vi "Measurement Logic.vi"(8 "error in":errorcluster, 9 "measurement configuration":T2={"Automation Test"=FALSE, "Power sequencing file path"="", "SMU name"="", "SMU channel"="0", "RFSG name"="5842_0", "RFSG port"="", "RFSG attenuation mode"=enum."Constant Attenuation", "RFSG external attenuation (dB)"=2.0, "RFSG s-parameters orientation"=enum."Port2 Towards DUT", "RFSG s2p file path"="", "RFmx name"="5842_0", "RFmx port"="", "RFmx attenuation mode"=enum."Constant Attenuation", "RFmx external attenuation (dB)"=1.2, "RFmx attenuation path name"="", "RFmx s-parameters orientation"=enum."Port2 Towards DUT", "RFmx attenuation s2p path name"="", "RFmx s2p file path"="", "Compression_Expected DUT Gain (dB)"=17.5, "Compression_Max Linear Range (dBm)"=-10.0, "Compression_Compression Point (dB)"=1.0, "Compression_Target Pin (dBm)"=1.0, "Compression_RFSG Frequency Start (Hz)"=10000000000.0, "Compression_RFSG Frequency Stop (Hz)"=18000000000.0, "Compression_RFSG Number of Frequency Step"=10, "Compression_RFSG Power Start (dBm)"=-20.0, "Compression_RFSG Power Stop(dBm)"=1.0, "Compression_RFSG Power Step Size (dB)"=4.0, "Compression_RBW (Hz)"=0.0, "Compression_RF Measurement Interval (s)"=0.0, "Compression_DC Measurement Interval (s)"=0.001, "Compression_Stimulus Mode"=enum."Constant Power and RF", "CP_CW_DC Source Delay (s)"=0.0, "CP_PRF_DC Source Delay (s)"=0.0, "CP_PRF_RFmx Trigger Delay (s)"=0.0, "CP_PRF_RF Pulse Width (s)"=0.0001, "CP_PRF_PRI (s)"=0.001, "PP_PRF_DC Source Delay (s)"=0.0, "PP_PRF_RFmx Trigger Delay (s)"=0.0, "PP_PRF_RF Pulse Width (s)"=0.0001, "PP_PRF_PRI (s)"=0.001, "PP_PRF_DC Pulse Width (s)"=0.0008, "PP_PRF_ON Current Limit (A)"=2.0, "PP_PRF_Bias Voltage Level (V)"=0.0, "PP_PRF_Bias Current Limit (A)"=0.2} {"Compression_Target Pin (dBm)" format="%#pdBm"; "PP_PRF_Bias Current Limit (A)" format="%#pA"; "PP_PRF_Bias Voltage Level (V)" format="%#pV"; "PP_PRF_ON Current Limit (A)" format="%#pA"; "PP_PRF_DC Pulse Width (s)" format="%#ps"; "PP_PRF_PRI (s)" format="%#ps"; "PP_PRF_RF Pulse Width (s)" format="%#ps"; "PP_PRF_RFmx Trigger Delay (s)" format="%#ps"; "PP_PRF_DC Source Delay (s)" format="%#ps"; "CP_PRF_PRI (s)" format="%#ps"; "CP_PRF_RF Pulse Width (s)" format="%#ps"; "CP_PRF_RFmx Trigger Delay (s)" format="%#ps"; "CP_PRF_DC Source Delay (s)" format="%#ps"; "CP_CW_DC Source Delay (s)" format="%#ps"; "Compression_DC Measurement Interval (s)" format="%#ps"; "Compression_RF Measurement Interval (s)" format="%#ps"; "RFmx external attenuation (dB)" format="%.2f"; "RFSG external attenuation (dB)" format="%.2f"}, 10 "measure call context in":refnum<class "Measure Call Context.lvclass">) -> (0 "error out":errorcluster, 1 "measurement results":T1, 2 "measure call context out":refnum<class "Measure Call Context.lvclass">)   [LabVIEW 2023, in "FPT_Compression.lvclass"]
doc: "Contains the core logic for executing the measurement."
uses:
  FPT_Compression.lvclass
  <vilib>/Plug-In SDKs/Measurements/Measure Call Context/Measure Call Context.lvclass
  Measurement Configuration.ctl
  Measurement Results.ctl
  <vilib>/Analysis/baseanly.llb/Mean (DBL).vi
  <extravilib>/ChannelInstances/Event Messenger-bool/Instantiate.vi
  <vilib>/Analysis/NI_AALBase.lvlib
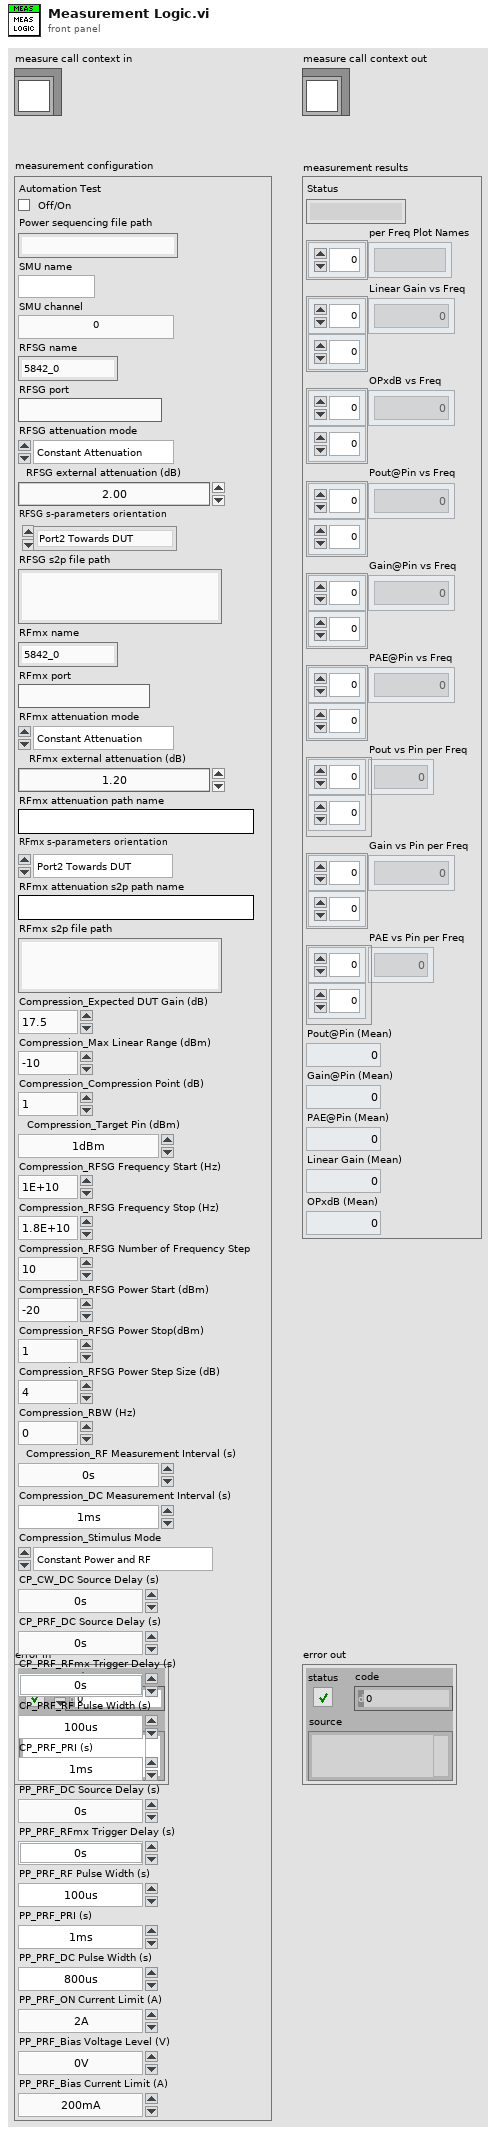
[diagram p1: front panel]
types:
  T1 = typedef "FPT_Compression.lvclass/Measurement Results.ctl" = cluster{"Status":string, "per Freq Plot Names":string[], "Linear Gain vs Freq":dbl[][], "OPxdB vs Freq":dbl[][], "Pout@Pin vs Freq":dbl[][], "Gain@Pin vs Freq":dbl[][], "PAE@Pin vs Freq":dbl[][], "Pout vs Pin per Freq":dbl[][], "Gain vs Pin per Freq":dbl[][], "PAE vs Pin per Freq":dbl[][], "Pout@Pin (Mean)":dbl, "Gain@Pin (Mean)":dbl, "PAE@Pin (Mean)":dbl, "Linear Gain (Mean)":dbl, "OPxdB (Mean)":dbl}
  T2 = typedef "FPT_Compression.lvclass/Measurement Configuration.ctl" = cluster{"Automation Test":bool, "Power sequencing file path":string, "SMU name":string, "SMU channel":string, "RFSG name":string, "RFSG port":string, "RFSG attenuation mode":enum32{"<None>", "Constant Attenuation", "s2p File"}, "RFSG external attenuation (dB)":dbl, "RFSG s-parameters orientation":enum32{"Port1 Towards DUT", "Port2 Towards DUT"}, "RFSG s2p file path":string, "RFmx name":string, "RFmx port":string, "RFmx attenuation mode":enum32{"<None>", "Constant Attenuation", "s2p File"}, "RFmx external attenuation (dB)":dbl, "RFmx attenuation path name":string, "RFmx s-parameters orientation":enum32{"Port1 Towards DUT", "Port2 Towards DUT"}, "RFmx attenuation s2p path name":string, "RFmx s2p file path":string, "Compression_Expected DUT Gain (dB)":dbl, "Compression_Max Linear Range (dBm)":dbl, "Compression_Compression Point (dB)":dbl, "Compression_Target Pin (dBm)":dbl, "Compression_RFSG Frequency Start (Hz)":dbl, "Compression_RFSG Frequency Stop (Hz)":dbl, "Compression_RFSG Number of Frequency Step":i32, "Compression_RFSG Power Start (dBm)":dbl, "Compression_RFSG Power Stop(dBm)":dbl, "Compression_RFSG Power Step Size (dB)":dbl, "Compression_RBW (Hz)":dbl, "Compression_RF Measurement Interval (s)":dbl, "Compression_DC Measurement Interval (s)":dbl, "Compression_Stimulus Mode":enum32{"Constant Power and RF", "Constant Power and Pulsed RF", "Pulsed Power and RF"}, "CP_CW_DC Source Delay (s)":dbl, "CP_PRF_DC Source Delay (s)":dbl, "CP_PRF_RFmx Trigger Delay (s)":dbl, "CP_PRF_RF Pulse Width (s)":dbl, "CP_PRF_PRI (s)":dbl, "PP_PRF_DC Source Delay (s)":dbl, "PP_PRF_RFmx Trigger Delay (s)":dbl, "PP_PRF_RF Pulse Width (s)":dbl, "PP_PRF_PRI (s)":dbl, "PP_PRF_DC Pulse Width (s)":dbl, "PP_PRF_ON Current Limit (A)":dbl, "PP_PRF_Bias Voltage Level (V)":dbl, "PP_PRF_Bias Current Limit (A)":dbl}
  T3 = enum32{"Power On Dut", "De-embedding + Measurement", "Power Off Dut"}[]
  T4 = cluster{"measurement configuration":T2, "measurement results":T1}
  T5 = typedef "RFmx Config - Compression.ctl" = cluster{"RFmx Name":refnum<k15>, "RFmx Port":string, "Attenuation":cluster{"Mode":enum32{"<None>", "Constant Attenuation", "s2p File"}, "Constant Attenuation":cluster{"RFmx External Attenuation (dB)":dbl}, "s2p File":cluster{"RFmx S-Parameters Orientation":i32, "RFmx Attenuation s2p File":path}}}
  T6 = typedef "RFSG Config - Compression.ctl" = cluster{"RFSG Name":refnum<k15>, "RFSG Port":string, "Attenuation":cluster{"Mode":enum32{"<None>", "Constant Attenuation", "s2p File"}, "Contant Attenuation":cluster{"RFSG External Attenuation (dB)":dbl}, "s2p File":cluster{"RFSG S-parameters Orientation":i32, "RFSG s2p File Path":path}}}
  T7 = typedef "Test Config - Compression.ctl" = cluster{"Expected DUT Gain (dB)":dbl, "Max Linear Range (dBm)":dbl, "Compression Point (dB)":dbl, "Pout at Pin (dBm)":dbl, "RFSG Frequency Start (Hz)":dbl, "RFSG Frequency Stop (Hz)":dbl, "RFSG Number of Frequency Step":i32, "Power Start (dBm)":dbl, "Power Stop(dBm)":dbl, "Power Step Size (dB)":dbl, "RBW (Hz)":dbl, "Modes":cluster{"RF Measurement Interval (s)":dbl, "DC Measurement Interval (s)":dbl, "Power Stimulus Mode":enum16{"Constant Power and RF", "Constant Power and Pulsed RF", "Pulsed Power and RF"}, "CP_CW_DC Source Delay (s)":dbl, "CP_PRF_RF Pulse Width (s)":dbl, "CP_PRF_PRI (s)":dbl, "CP_PRF_DC Source Delay (s)":dbl, "CP_PRF_RFmx Trigger Delay (s)":dbl, "PP_PRF_RF Pulse Width (s)":dbl, "PP_PRF_PRI (s)":dbl, "PP_PRF_DC Pulse Width (s)":dbl, "PP_PRF_Bias Voltage Level (V)":dbl, "PP_PRF_Bias Current Limit (A)":dbl, "PP_PRF_DC Source Delay (s)":dbl, "PP_PRF_RFmx Trigger Delay (s)":dbl}}
  T8 = typedef "SMU Config - Compression.ctl" = cluster{"SMU Name":refnum<k15>, "SMU Channel":string, "IDD Current Limit (A)":dbl}
  T9 = typedef "Results - Compression.ctl" = cluster{"Linear Gain vs Freq":dbl[][], "OPxdb vs Freq":dbl[][], "Pout@Pin vs Freq":dbl[][], "Gain@Pin vs Freq":dbl[][], "PAE@Pin vs Freq":dbl[][], "Pout vs Pin per Freq":dbl[][], "Gain vs Pin per Freq":dbl[][], "PAE vs Pin per Freq":dbl[][]}
  T10 = typedef "Event Messenger-bool.lvlib/))Channel.ctl" = refnum<queue>
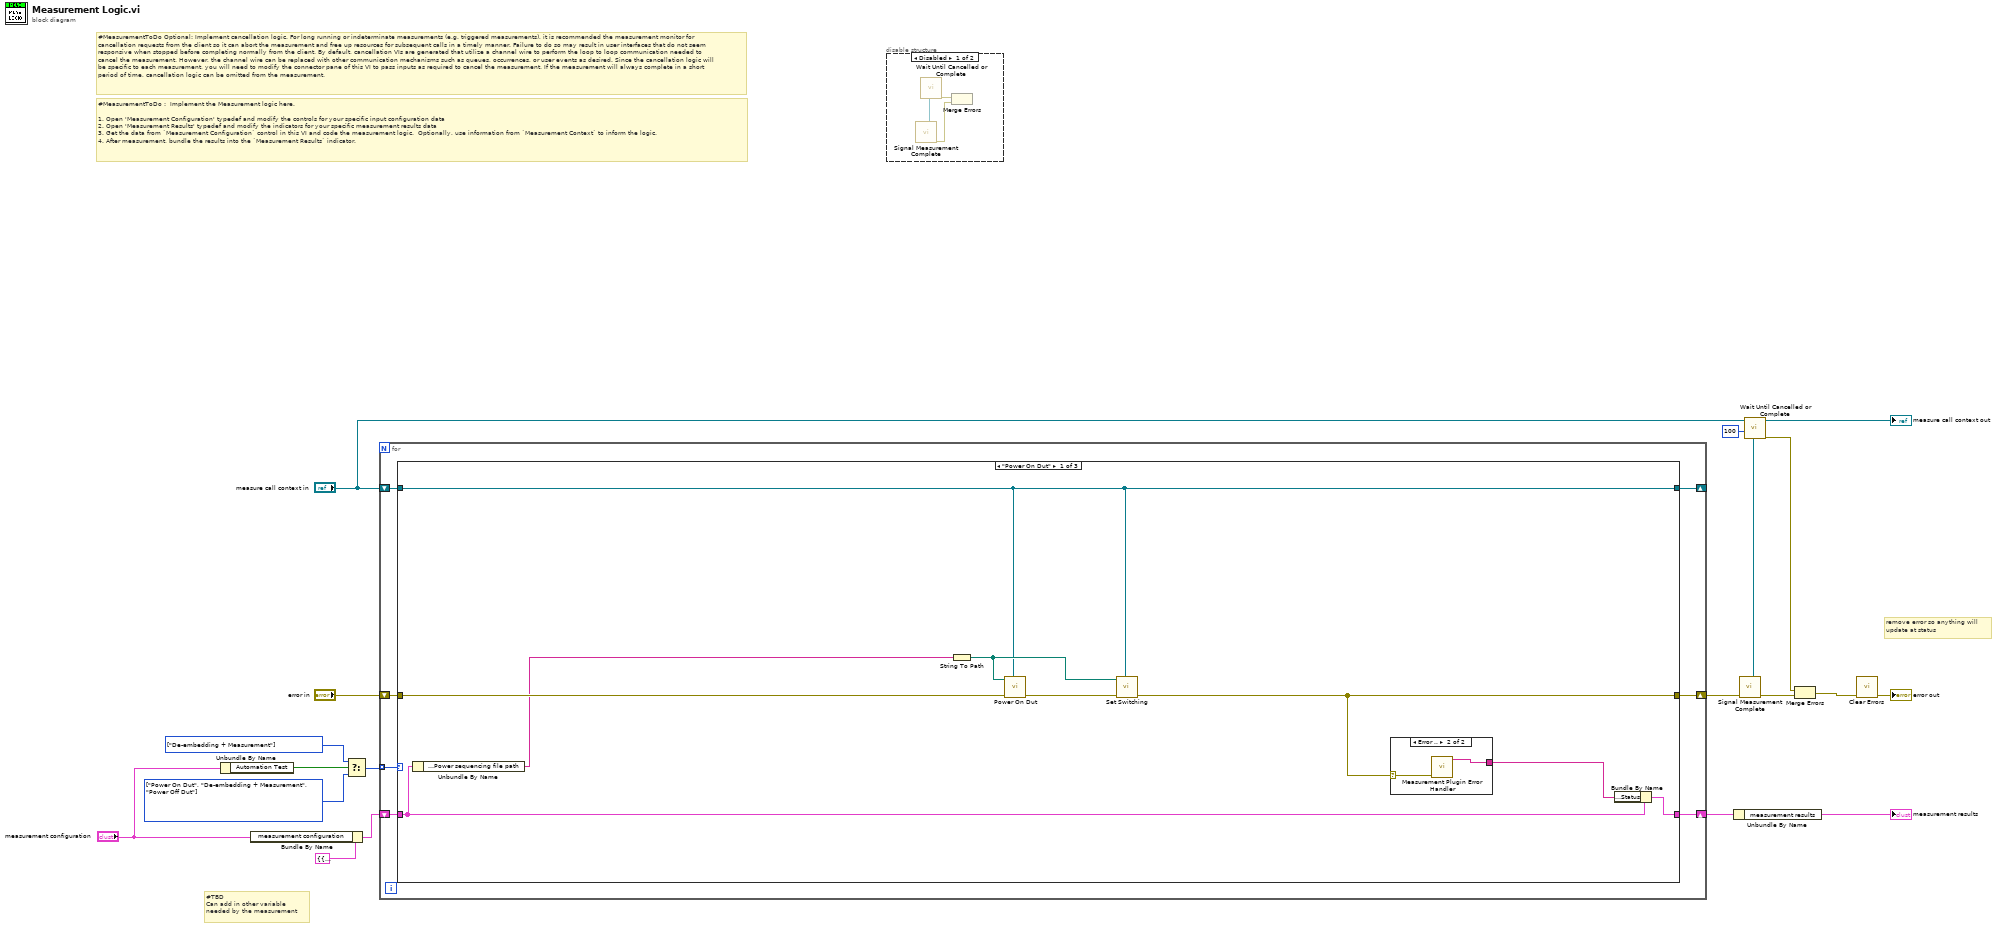
[diagram p0: block diagram]
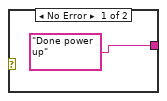
[diagram p2: hidden frame]
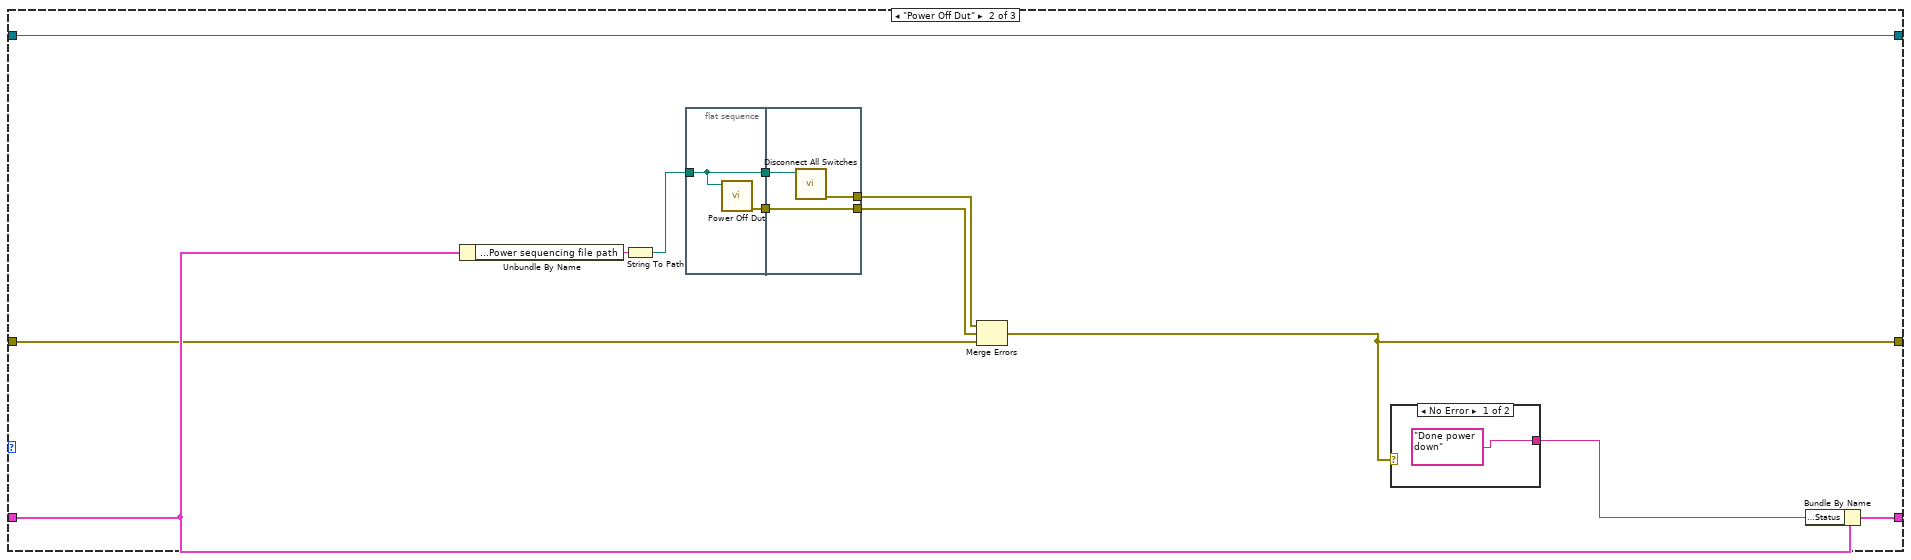
[diagram p3: hidden frame]
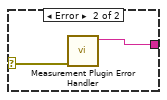
[diagram p4: hidden frame]
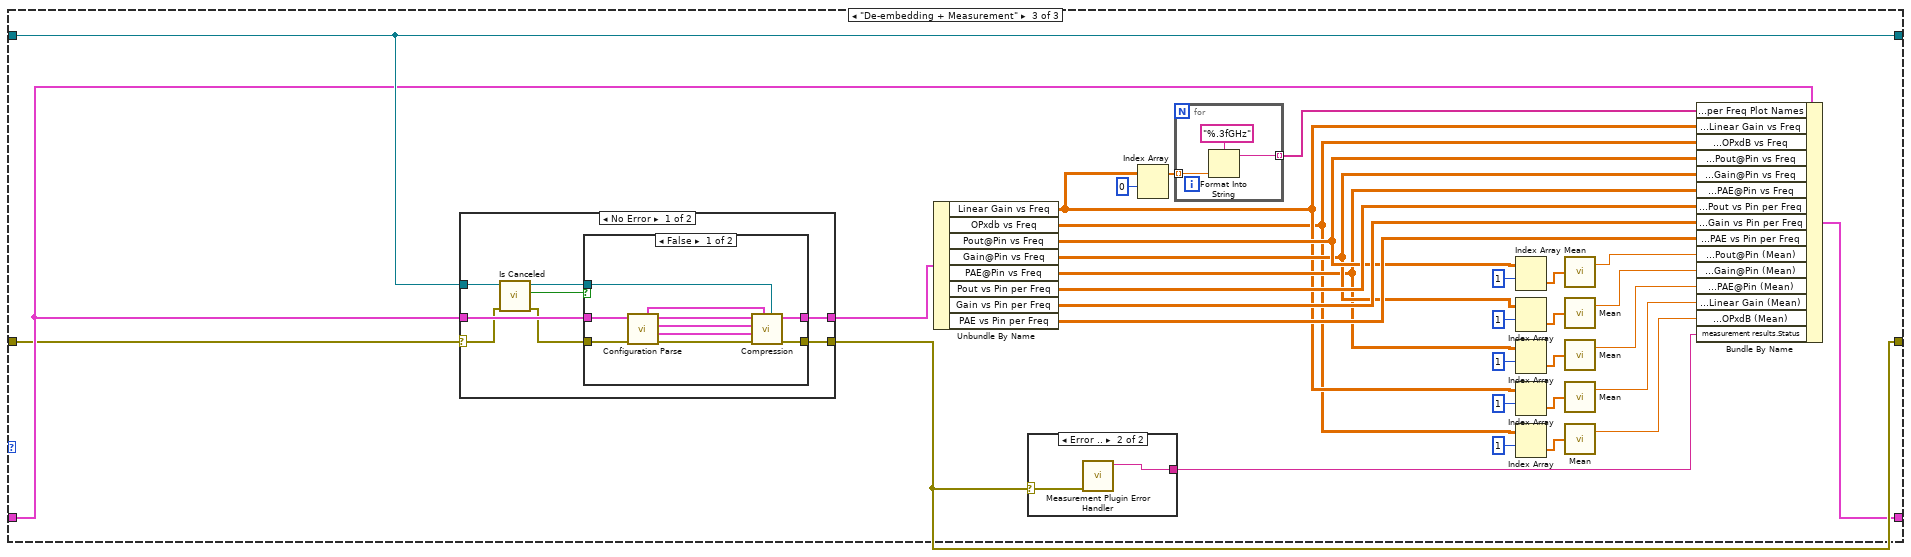
[diagram p5: hidden frame]
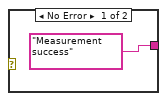
[diagram p8: hidden frame]
diagram:
  w12 = T3 [enum."De-embedding + Measurement"] items=["Power On Dut", "De-embedding + Measurement", "Power Off Dut"]
  w14 = T3 [enum."Power On Dut", enum."De-embedding + Measurement", enum."Power Off Dut"] items=["Power On Dut", "De-embedding + Measurement", "Power Off Dut"]
  # "remove error so anything will\nupdate at status"
  # "#TBD\nCan add in other variable\nneeded by the measurement"
  # "#MeasurementToDo Optional: Implement cancellation logic. For long running or indeterminate measurements (e.g. triggered measurements), it is recommended the measurement monitor for cancellation requests from the client so it can abort the measurement and free up resources for subsequent calls in a timely manner. Failure to do so may result in user interfaces that do not seem responsive when stopped before completing normally from the client. By default, cancellation VIs are generated that utilize a channel wire to perform the loop to loop communication needed to cancel the measurement. However, the channel wire can be replaced with other communication mechanisms such as queues, occurrences, or user events as desired. Since the cancellation logic will be specific to each measurement, you will need to modify the connector pane of this VI to pass inputs as required to cancel the measurement. If the measurement will always complete in a short period of time, cancellation logic can be omitted from the measurement."
  # "#MeasurementToDo :  Implement the Measurement logic here.\n\n1. Open 'Measurement Configuration' typedef and modify the controls for your specific input configuration data\n2. Open 'Measurement Results' typedef and modify the indicators for your specific measurement results data\n3. Get the data from `Measurement Configuration` control in this VI and code the measurement logic.  Optionally, use information from `Measurement Context` to inform the logic.\n4. After measurement, bundle the results into the `Measurement Results` indicator."
  n1 = Unbundle By Name("measurement configuration") -> ("Automation Test"=w10:bool)
  n2 = Bundle By Name(cluster=T4 {"measurement configuration"={"Automation Test"=FALSE, "Power sequencing file path"="", "SMU name"="", "SMU channel"="0", "RFSG name"="5842_0", "RFSG port"="", "RFSG attenuation mode"=enum."Constant Attenuation", "RFSG external attenuation (dB)"=2.0, "RFSG s-parameters orientation"=enum."Port2 Towards DUT", "RFSG s2p file path"="", "RFmx name"="5842_0", "RFmx port"="", "RFmx attenuation mode"=enum."Constant Attenuation", "RFmx external attenuation (dB)"=1.2, "RFmx attenuation path name"="", "RFmx s-parameters orientation"=enum."Port2 Towards DUT", "RFmx attenuation s2p path name"="", "RFmx s2p file path"="", "Compression_Expected DUT Gain (dB)"=17.5, "Compression_Max Linear Range (dBm)"=-10.0, "Compression_Compression Point (dB)"=1.0, "Compression_Target Pin (dBm)"=1.0, "Compression_RFSG Frequency Start (Hz)"=10000000000.0, "Compression_RFSG Frequency Stop (Hz)"=18000000000.0, "Compression_RFSG Number of Frequency Step"=10, "Compression_RFSG Power Start (dBm)"=-20.0, "Compression_RFSG Power Stop(dBm)"=1.0, "Compression_RFSG Power Step Size (dB)"=4.0, "Compression_RBW (Hz)"=0.0, "Compression_RF Measurement Interval (s)"=0.0, "Compression_DC Measurement Interval (s)"=0.001, "Compression_Stimulus Mode"=enum."Constant Power and RF", "CP_CW_DC Source Delay (s)"=0.0, "CP_PRF_DC Source Delay (s)"=0.0, "CP_PRF_RFmx Trigger Delay (s)"=0.0, "CP_PRF_RF Pulse Width (s)"=0.0001, "CP_PRF_PRI (s)"=0.001, "PP_PRF_DC Source Delay (s)"=0.0, "PP_PRF_RFmx Trigger Delay (s)"=0.0, "PP_PRF_RF Pulse Width (s)"=0.0001, "PP_PRF_PRI (s)"=0.001, "PP_PRF_DC Pulse Width (s)"=0.0008, "PP_PRF_ON Current Limit (A)"=2.0, "PP_PRF_Bias Voltage Level (V)"=0.0, "PP_PRF_Bias Current Limit (A)"=0.2}, "measurement results"={"Status"="", "per Freq Plot Names"=[], "Linear Gain vs Freq"=[], "OPxdB vs Freq"=[], "Pout@Pin vs Freq"=[], "Gain@Pin vs Freq"=[], "PAE@Pin vs Freq"=[], "Pout vs Pin per Freq"=[], "Gain vs Pin per Freq"=[], "PAE vs Pin per Freq"=[], "Pout@Pin (Mean)"=0.0, "Gain@Pin (Mean)"=0.0, "PAE@Pin (Mean)"=0.0, "Linear Gain (Mean)"=0.0, "OPxdB (Mean)"=0.0}}, "measurement configuration"="measurement configuration") -> (w18:T4)
  n3 = Select(t=w12, s=w10, f=w14) -> (s? t:f=w13:T3)
  n4 = for {
    tunnel: w13 -> [w25] mode=indexing
    shift-right: [w20] -> w8
    shift-left: "error in" -> [w26]
    shift-right: [w21] -> w17
    shift-left: w18 -> [w24]
    shift-right: [w22] -> _
    shift-left: "measure call context in" -> [w23]
    n5 = case shown="\"Power On Dut\"" w25 {
      tunnel: w26 -> [w35 w41 w59]
      tunnel: w24 -> [w34 w47 w60]
      tunnel: w23 -> [w27 w42 w89]
      tunnel: [w28 w43 w91] -> w20
      tunnel: [w27 w42 w89] -> w22
      tunnel: [w32 w48 w90] -> w21
      frame "Power On Dut" {
        n6 = Unbundle By Name(w34) -> ("measurement configuration.Power sequencing file path"=w31:string)
        n7 = String To Path(string=w31) -> (path=w29:path)
        n8 = call "Power On Dut.vi"("measure call context in"=w27, "error in"=w35, "Power sequencing file path"=w29) -> ("error out"=w30:errorcluster)  [unwired: 7 in, 1 out]
        n9 = call "Set Switching.vi"("measure call context in"=w27, "error in"=w30, "File Path"=w29) -> ("error out"=w28:errorcluster)  [unwired: 7 in, 1 out]
        n10 = case shown="Error .." w28 {
          selector: w28 -> [_ w38]
          tunnel: ["Done power up" w37] -> w33
          frame No Error {
          }
          frame Error {
            n11 = call "Measurement Plugin Error Handler.vi"("error in"=w38) -> ("Status Message (Error)"=w37:string)  [unwired: 9 in, 1 out]
          }
        }
        n12 = Bundle By Name(cluster=w34, "measurement results.Status"=w33) -> (w32:T4)
      }
      frame "Power Off Dut" {
        n13 = Unbundle By Name(w47) -> ("measurement configuration.Power sequencing file path"=w50:string)
        n14 = String To Path(string=w50) -> (path=w45:path)
        n15 = flat-sequence {
          tunnel: w45 -> [w54]
          tunnel: [w55] -> w46
          tunnel: [w54] -> w44
          tunnel: w46 -> [w58]
          tunnel: w44 -> [w56]
          tunnel: [w58] -> w39
          tunnel: [w57] -> w40
          frame #0 {
            n16 = call "Power Off Dut.vi"("Power Sequencing File Path"=w54) -> ("error out"=w55:errorcluster)  [unwired: 10 in]
          }
          frame #1 {
            n17 = call "Disconnect All Switches.vi"("File Path"=w56) -> ("error out"=w57:errorcluster)  [unwired: 10 in]
          }
        }
        n18 = Merge Errors(w40, w39, w41) -> (w43:errorcluster)
        n19 = case shown="No Error" w43 {
          selector: w43 -> [_ w53]
          tunnel: ["Done power down" w52] -> w49
          frame No Error {
          }
          frame Error {
            n20 = call "Measurement Plugin Error Handler.vi"("error in"=w53) -> ("Status Message (Error)"=w52:string)  [unwired: 9 in, 1 out]
          }
        }
        n21 = Bundle By Name(cluster=w47, "measurement results.Status"=w49) -> (w48:T4)
      }
      frame "De-embedding + Measurement" {
        n22 = case shown="No Error" w59 {
          selector: w59 -> [w93 w111]
          tunnel: [w99 w111] -> w91
          tunnel: w89 -> [w95 _]
          tunnel: [w98 _] -> w81
          tunnel: w60 -> [w97 _]
          frame No Error {
            n23 = call <vilib>:"Is Canceled.vi"("error in"=w93, "measure call context in"=w95) -> ("error out"=w92:errorcluster, "is canceled?"=w96:bool, "measure call context out"=w94:refnum<class "Measure Call Context.lvclass">)  [unwired: 7 in]
            n24 = case shown="False" w96 {
              tunnel: [w109 w110] -> w99
              tunnel: w94 -> [w108 _]
              tunnel: [w107 _] -> w98
              tunnel: w97 -> [w106 _]
              tunnel: w92 -> [w105 w110]
              frame False {
                n25 = call "Configuration Parse.vi"("error in"=w105, "UI Controls"=w106) -> ("error out"=w101:errorcluster, "RFmx Settings"=w102:T5, "RFSG Settings"=w103:T6, "Test Configuration"=w104:T7, "SMU Settings"=w100:T8)  [unwired: 5 in]
                n26 = call "Compression.vi"("measure call context in"=w108, "SMU Settings"=w100, "error in"=w101, "RFmx Settings"=w102, "RFSG Settings"=w103, "Test Configuration"=w104) -> ("error out"=w109:errorcluster, "Data"=w107:T9)  [unwired: 4 in]
              }
              frame True {
                # "Canceled"
              }
            }
          }
          frame Error {
          }
        }
        n27 = Unbundle By Name(w81) -> ("Linear Gain vs Freq"=w67:dbl[][], "OPxdb vs Freq"=w64:dbl[][], "Pout@Pin vs Freq"=w73:dbl[][], "Gain@Pin vs Freq"=w72:dbl[][], "PAE@Pin vs Freq"=w71:dbl[][], "Pout vs Pin per Freq"=w80:dbl[][], "Gain vs Pin per Freq"=w79:dbl[][], "PAE vs Pin per Freq"=w78:dbl[][])
        n28 = case shown="Error .." w91 {
          selector: w91 -> [_ w114]
          tunnel: ["Measurement success" w113] -> w61
          frame No Error {
          }
          frame Error {
            n29 = call "Measurement Plugin Error Handler.vi"("error in"=w114) -> ("Status Message (Error)"=w113:string)  [unwired: 9 in, 1 out]
          }
        }
        n30 = Index Array(array=w67, index (row)=0) -> (element=w85:dbl[])  [unwired: 1 in]
        n31 = for {
          tunnel: w85 -> [w115] mode=indexing
          tunnel: [w116] -> w83 mode=indexing
          # "Get Plot Names"
          n32 = Format Into String(format string="%.3fGHz", w115) -> (resulting string=w116:string)  [unwired: 2 in, 1 out]
        }
        n33 = Index Array(array=w73, index (row)=1) -> (element=w77:dbl[])  [unwired: 1 in]
        n34 = Index Array(array=w72, index (row)=1) -> (element=w74:dbl[])  [unwired: 1 in]
        n35 = Index Array(array=w71, index (row)=1) -> (element=w76:dbl[])  [unwired: 1 in]
        n36 = Index Array(array=w67, index (row)=1) -> (element=w75:dbl[])  [unwired: 1 in]
        n37 = Index Array(array=w64, index (row)=1) -> (element=w66:dbl[])  [unwired: 1 in]
        n38 = call-poly <vilib>:"Mean.vi"("X"=w77) -> ("mean"=w70:dbl)  [unwired: 1 out]
        n39 = call-poly <vilib>:"Mean.vi"("X"=w74) -> ("mean"=w69:dbl)  [unwired: 1 out]
        n40 = call-poly <vilib>:"Mean.vi"("X"=w76) -> ("mean"=w68:dbl)  [unwired: 1 out]
        n41 = call-poly <vilib>:"Mean.vi"("X"=w75) -> ("mean"=w63:dbl)  [unwired: 1 out]
        n42 = call-poly <vilib>:"Mean.vi"("X"=w66) -> ("mean"=w62:dbl)  [unwired: 1 out]
        n43 = Bundle By Name(cluster=w60, "measurement results.per Freq Plot Names"=w83, "measurement results.Linear Gain vs Freq"=w67, "measurement results.OPxdB vs Freq"=w64, "measurement results.Pout@Pin vs Freq"=w73, "measurement results.Gain@Pin vs Freq"=w72, "measurement results.PAE@Pin vs Freq"=w71, "measurement results.Pout vs Pin per Freq"=w80, "measurement results.Gain vs Pin per Freq"=w79, "measurement results.PAE vs Pin per Freq"=w78, "measurement results.Pout@Pin (Mean)"=w70, "measurement results.Gain@Pin (Mean)"=w69, "measurement results.PAE@Pin (Mean)"=w68, "measurement results.Linear Gain (Mean)"=w63, "measurement results.OPxdB (Mean)"=w62, "measurement results.Status"=w61) -> (w90:T4)
      }
    }
  }
  n44 = disable-structure shown="Disabled" {
    frame Disabled {
      n45 = call "Signal Measurement Complete.vi"() -> ("error out"=w119:errorcluster, "done channel"=w120:T10)  [unwired: 10 in]
      n46 = call "Wait Until Cancelled or Complete.vi"("done channel"=w120) -> ("error out"=w118:errorcluster)  [unwired: 9 in, 1 out]
      n47 = Merge Errors(w118, w119) -> ()  [unwired: 1 out]
    }
    frame Enabled {
    }
  }
  n48 = Unbundle By Name(w17) -> ("measurement results"=→"measurement results":T1)
  n49 = call "Signal Measurement Complete.vi"("error in (no error)"=w8) -> ("error out"=w7:errorcluster, "done channel"=w6:T10)  [unwired: 9 in]
  n50 = call "Wait Until Cancelled or Complete.vi"("done channel"=w6, "ms polling interval"=100, "measure call context in"="measure call context in") -> ("error out"=w2:errorcluster, "measure call context out"=→"measure call context out":refnum<class "Measure Call Context.lvclass">)  [unwired: 7 in]
  n51 = Merge Errors(w2, w7) -> (w4:errorcluster)
  n52 = call <vilib>:"Clear Errors.vi"("error in (no error)"=w4) -> ("error out"=→"error out":errorcluster)  [unwired: 5 in, 1 out]
